vi "Bare_Minimum.vi"() -> ()   [LabVIEW 2014]
uses:
  <userlib>/UCSD Robotics Lab/Robotics-Cape/LV/libroboticscape.lvlib
panel:
  out "Timing Block":T1 {"Actual Hz" format="%#_3g"; "Dt" format="%#_4g"; "Average Hz" format="%#_4g"}
  out "Iteration counter":i32
  out "State":T2(ring)
  in  "stop":bool
  # "Always stop the VI using the rectangular STOP button above, never with the round stopsign (Abort)"
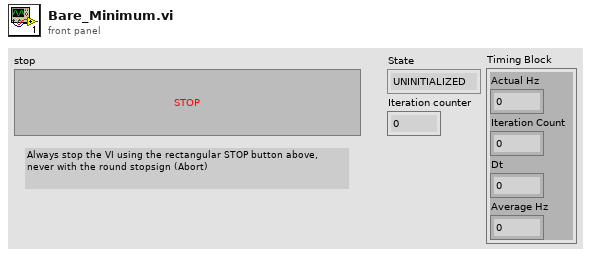
[diagram p1: front panel]
types:
  T1 = cluster{"Actual Hz":dbl, "Iteration Count":dbl, "Dt":dbl, "Average Hz":dbl}
  T2 = enum16{"UNINITIALIZED", "RUNNING", "PAUSED", "EXITING"}
  T3 = enum16{"UNINITIALIZED", "RUNING", "PAUSED", "EXITING"}
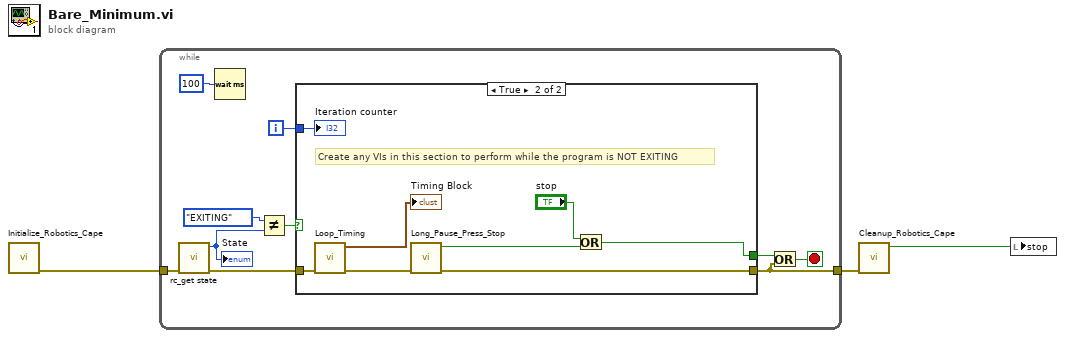
[diagram p0: block diagram]
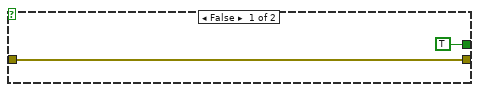
[diagram p2: hidden frame]
diagram:
  n1 = call "Initialize_Robotics_Cape.vi"() -> ("error out"=w3:errorcluster)  [unwired: 11 in]
  n2 = while {
    tunnel: w3 -> [w12]
    tunnel: [w6] -> w2
    i -> [w11]
    stop <- w13 stop-if-true
    n3 = call <userlib>:"rc_get state.vi"("error in (no error)"=w12) -> ("error out"=w7:errorcluster, "function return"=w9:u32)  [unwired: 9 in]
    "State" <- w9
    n4 = Wait (ms)(milliseconds to wait=u32 100) -> ()  [unwired: 1 out]
    n5 = Not Equal?(x=T3."EXITING" ("State 2"), y=w9) -> (x != y?=w8:bool)
    n6 = case shown="True" w8 {
      tunnel: w11 -> [_ w23]
      tunnel: w7 -> [w15 w22]
      tunnel: [w15 w19] -> w6
      tunnel: [TRUE ("stop") w16] -> w5
      frame False {
      }
      frame True {
        # "Create any VIs in this section to perform while the program is NOT EXITING"
        n7 = call "Loop_Timing.vi"("error in"=w22) -> ("error out"=w20:errorcluster, "Timing Block"=→"Timing Block":T1)  [unwired: 9 in]
        n8 = call "Long_Pause_Press_Stop.vi"("error in (no error)"=w20) -> ("error out"=w19:errorcluster, "Stop"=w18:bool)  [unwired: 9 in]
        n9 = Or(x="stop", y=w18) -> (x .or. y?=w16:bool)
        "Iteration counter" <- w23
      }
    }
    n10 = Or(x=w5, y=w6) -> (x .or. y?=w13:bool)
  }
  n11 = call "Cleanup_Robotics_Cape.vi"("error in (no error)"=w2) -> ("Stop Local Variabl"=w1:bool)  [unwired: 9 in, 1 out]
  n12 = local write "stop"(w1) -> ()
